vi "Zad2.vi"() -> ()   [LabVIEW 2017]
uses:
  Lab 6 - 9.04.2018/mainVIs/States.ctl
  <vilib>/sound2/lvsound2.llb/Sound Data Format.ctl
  <vilib>/sound2/lvsound2.llb/Sound Input Task ID.ctl
  <vilib>/sound2/lvsound2.llb/Sampling Mode.ctl
  <vilib>/measure/maspectr.llb/FFT Power Spectrum and PSD for N Chan.vi
  <vilib>/sound2/lvsound2.llb/Sound Input Read (DBL).vi
  <vilib>/measure/NI_MAPro.lvlib
panel:
  out "Waveform Graph":cluster{"f0":dbl, "df":dbl, "magnitude":dbl[]}[](graph)
  in  "stop":bool
  in  "Play":bool
  in  "sound format":T1={"sample rate (S/s)"=22050.0, "number of channels"=2, "bits per sample"=16}
  in  "number of samples/ch":i32=100000
  out "Enum":T2
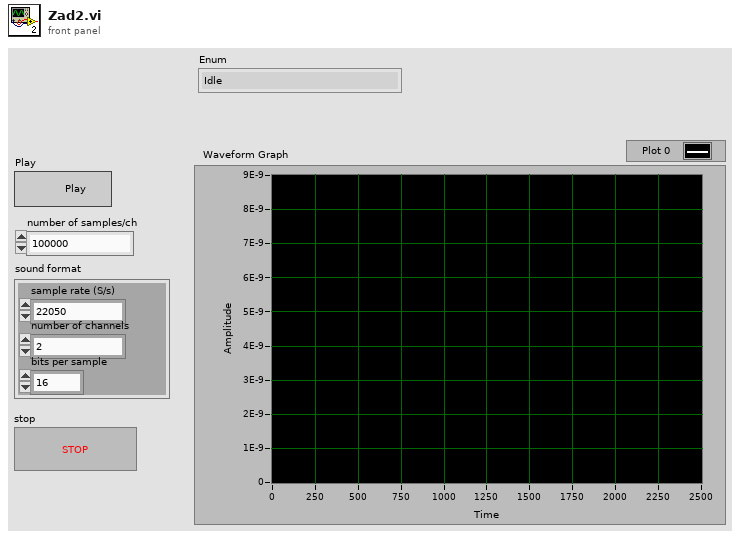
[diagram p1: front panel]
types:
  T1 = typedef "Sound Data Format.ctl" = cluster{"sample rate (S/s)":dbl, "number of channels":i32, "bits per sample":i32}
  T2 = typedef "States.ctl" = enum16{"Idle", "Initialization", "Acquisition", "Finish"}
  T3 = typedef "Sound Input Task ID.ctl" = u32
  T4 = typedef "Sampling Mode.ctl" = i32
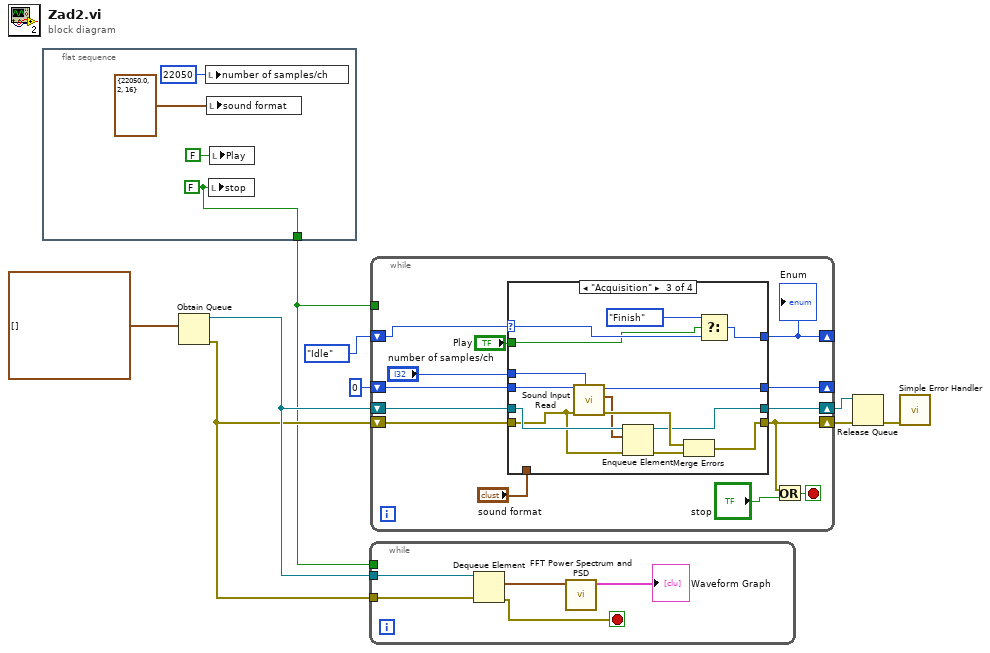
[diagram p0: block diagram]
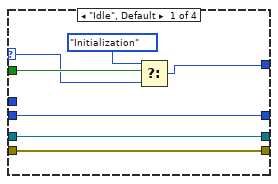
[diagram p2: hidden frame]
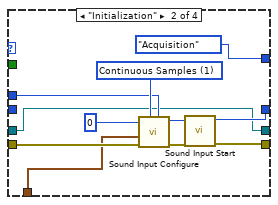
[diagram p3: hidden frame]
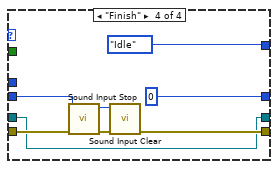
[diagram p4: hidden frame]
diagram:
  n1 = flat-sequence {
    tunnel: [w11] -> w1
    frame #0 {
      w11 = FALSE ("stop")
      n2 = local write "number of samples/ch"(22050 ("number of samples/ch")) -> ()
      n3 = local write "sound format"(T1 {"sample rate (S/s)"=22050.0, "number of channels"=2, "bits per sample"=16} ("sound format")) -> ()
      n4 = local write "stop"(w11) -> ()
      n5 = local write "Play"(FALSE ("Play")) -> ()
    }
  }
  n6 = Obtain Queue(element data type=waveform(dbl)[] [] ("data")) -> (queue out=w4:refnum<queue>, error out=w3:errorcluster)  [unwired: 4 in, 1 out]
  n7 = while {
    tunnel: w4 -> [w18]
    tunnel: w3 -> [w17]
    tunnel: w1 -> [_]
    stop <- w16 stop-if-true
    n8 = Dequeue Element(queue=w18, error in (no error)=w17) -> (element=w15:waveform(dbl)[], error out=w16:errorcluster)  [unwired: 1 in, 2 out]
    n9 = call-poly <vilib>:"FFT Power Spectrum and PSD.vi"("time signals"=w15) -> ("Power Spectrum / PSD"=→"Waveform Graph":cluster{"f0":dbl, "df":dbl, "magnitude":dbl[]}[])  [unwired: 7 in, 3 out]
  }
  n10 = while {
    shift-right: [w30] -> _
    shift-left: States."Idle" ("Enum") -> [w31]
    shift-right: [w22] -> w6
    shift-left: w3 -> [w28]
    shift-right: [w25] -> _
    shift-left: T3 0 ("task ID out") -> [w24]
    shift-right: [w19] -> w7
    shift-left: w4 -> [w20]
    tunnel: w1 -> [_]
    stop <- w23 stop-if-true
    n11 = case shown="\"Acquisition\"" w31 {
      selector: w31 -> [w35 _ w59 _]
      tunnel: [w38 States."Acquisition" ("Enum") w63 States."Idle" ("Enum")] -> w30
      tunnel: "Play" -> [w36 _ w57 _]
      tunnel: [w33 w42 w52 w66] -> w22
      tunnel: w28 -> [w33 w48 w55 w69]
      tunnel: "sound format" -> [_ w47 _ _]
      tunnel: "number of samples/ch" -> [_ w45 w60 _]
      tunnel: [w34 w41 w61 T3 0 ("task ID out")] -> w25
      tunnel: w24 -> [w34 _ w62 w70]
      tunnel: w20 -> [w32 w39 w56 w64]
      tunnel: [w32 w39 w51 w64] -> w19
      frame "Idle", Default {
        n12 = Select(t=States."Initialization" ("Enum"), s=w36, f=w35) -> (s? t:f=w38:T2)
      }
      frame "Initialization" {
        w46 = T4 1 items=["Finite Samples", "Continuous Samples"] ("sample mode")
        n13 = call <vilib>:"Sound Input Configure.vi"("number of samples/ch"=w45, "sample mode"=w46, "error in (no error)"=w48, "sound format"=w47, "device ID"=u32 0) -> ("error out"=w43:errorcluster, "task ID"=w44:T3)  [unwired: 5 in]
        n14 = call <vilib>:"Sound Input Start.vi"("error in (no error)"=w43, "task ID"=w44) -> ("error out"=w42:errorcluster, "task ID out"=w41:T3)  [unwired: 8 in]
      }
      frame "Acquisition" {
        n15 = call-poly <vilib>:"Sound Input Read.vi"("number of samples/ch"=w60, "error in (no error)"=w55, "task ID"=w62) -> ("error out"=w53:errorcluster, "data"=w50:waveform(dbl)[], "task ID out"=w61:T3)  [unwired: 6 in]
        n16 = Enqueue Element(queue=w56, element=w50, error in (no error)=w55) -> (queue out=w51:refnum<queue>, error out=w54:errorcluster)  [unwired: 1 in, 1 out]
        n17 = Merge Errors(w53, w54) -> (w52:errorcluster)
        n18 = Select(t=States."Finish" ("Enum"), s=w57, f=w59) -> (s? t:f=w63:T2)
      }
      frame "Finish" {
        n19 = call <vilib>:"Sound Input Stop.vi"("error in (no error)"=w69, "task ID"=w70) -> ("error out"=w67:errorcluster, "task ID out"=w68:T3)  [unwired: 8 in]
        n20 = call <vilib>:"Sound Input Clear.vi"("error in (no error)"=w67, "task ID"=w68) -> ("error out"=w66:errorcluster)  [unwired: 9 in]
      }
    }
    "Enum" <- w30
    n21 = Or(x=w22, y="stop") -> (x .or. y?=w23:bool)
  }
  n22 = Release Queue(queue=w7, error in (no error)=w6) -> (error out=w5:errorcluster)  [unwired: 1 in, 2 out]
  n23 = call <vilib>:"Simple Error Handler.vi"("error in (no error)"=w5) -> ()  [unwired: 4 in, 5 out]
